vi "Set Visibility of Select Manual Controls.vi"(9 "Visible (F)":bool, 10 "Control Names":string[](array[string])=["P Setpoint (kW)", "Write P", "Write Mode", "Gen Mode", "Write Q", "Q Setpoint (kVAR)"], 11 "VI in":refnum<vi>) -> ()   [LabVIEW 2018, in "EMS User Interface Actor.lvlib" / "EMS User Interface.lvclass"]
uses:
  EMS User Interface.lvclass
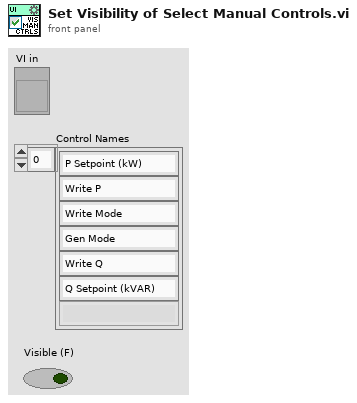
[diagram p1: front panel]
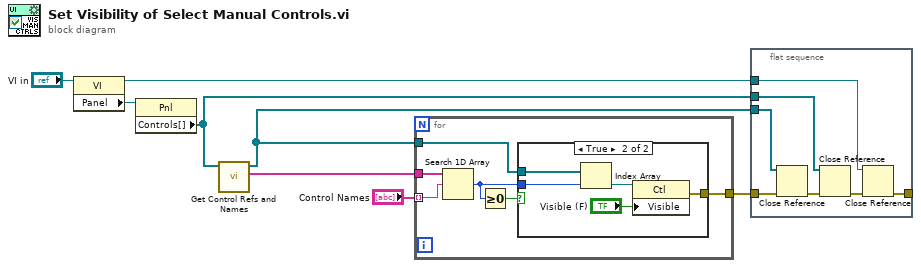
[diagram p0: block diagram]
diagram:
  n1 = property class="VI"(reference="VI in") -> (reference out=w8:refnum<vi>, "Panel"=w5:refnum<vi>)  [unwired: 1 in, 1 out]
  n2 = property class="Pnl"(reference=w5) -> ("Controls[]"=w3:refnum<vi>[])  [unwired: 1 in, 2 out]
  n3 = call "Get Control Refs and Names.vi"("Controls[]"=w3) -> ("Ctrl Labels"=w2:string[], "Ctrl Refs"=w1:refnum<vi>[])  [unwired: 9 in]
  n4 = for {
    tunnel: w2 -> [w14]
    tunnel: "Control Names" -> [w13] mode=indexing
    tunnel: w1 -> [w11]
    tunnel: [w9] -> w7
    n5 = Search 1D Array(1D array=w14, element=w13) -> (index of element=w10:i32)  [unwired: 1 in]
    n6 = Greater Or Equal To 0?(x=w10) -> (x >= 0?=w12:bool)
    n7 = case shown="True" w12 {
      tunnel: w11 -> [_ w19]
      tunnel: w10 -> [_ w18]
      tunnel: [_ w16] -> w9
      frame False {
      }
      frame True {
        n8 = Index Array(array=w19, index=w18) -> (element=w17:refnum<vi>)
        n9 = property class="Ctl"(reference=w17, "Visible"="Visible (F)") -> (error out=w16:errorcluster)  [unwired: 1 in, 1 out]
      }
    }
  }
  n10 = flat-sequence {
    tunnel: w7 -> [w22]
    tunnel: w3 -> [w26]
    tunnel: w8 -> [w24]
    tunnel: [w23] -> _
    tunnel: w1 -> [w20]
    frame #0 {
      n11 = Close Reference(reference=w20, error in (no error)=w22) -> (error out=w21:errorcluster)
      n12 = Close Reference(reference=w26, error in (no error)=w21) -> (error out=w25:errorcluster)
      n13 = Close Reference(reference=w24, error in (no error)=w25) -> (error out=w23:errorcluster)
    }
  }
